vi "Windows.SetCurrent App as Front Window.vi"(10 "Win Name":string, 11 "VI Ref":refnum<vi>) -> ()   [LabVIEW 2019]
uses:
  user32.dll
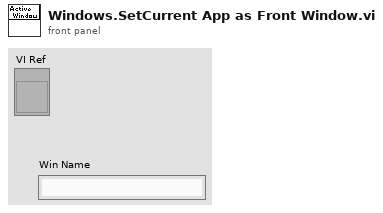
[diagram p1: front panel]
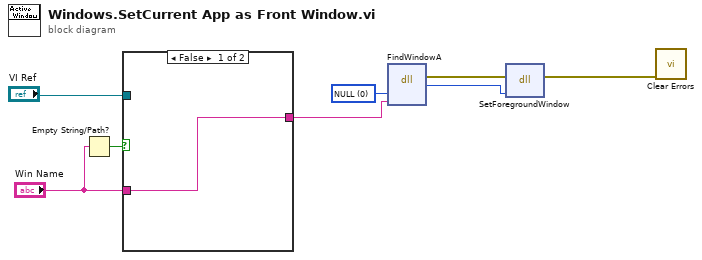
[diagram p0: block diagram]
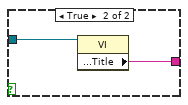
[diagram p2: hidden frame]
diagram:
  w8 = 0 items=["NULL"]
  n1 = Empty String/Path?(string/path="Win Name") -> (empty?=w2:bool)
  n2 = case shown="False" w2 {
    tunnel: [w9 w11] -> w5
    tunnel: "VI Ref" -> [_ w10]
    tunnel: "Win Name" -> [w9 _]
    frame False {
    }
    frame True {
      n3 = property class="VI"(reference=w10) -> ("Front Panel.Title"=w11:string)  [unwired: 1 in, 2 out]
    }
  }
  n4 = dll-call lib="user32.dll" fn="FindWindowA" label="FindWindow"("lpszClassName"=w8, "lpszWindowName"=w5) -> (error out=w6:errorcluster, "hWnd"=w7:u32)  [unwired: 4 in, 2 out]
  n5 = dll-call lib="user32.dll" fn="SetForegroundWindow"(error in=w6, "Handle"=w7) -> (error out=w3:errorcluster)  [unwired: 3 in, 2 out]
  n6 = call <vilib>:"Clear Errors.vi"("error in (no error)"=w3) -> ()  [unwired: 5 in, 2 out]
